vi "Microwave Amplifier Control Panel.vi"() -> ()   [LabVIEW 2009]
panel:
  in  "?":bool
  in  "?":bool
  out "Gain":dbl
  out "Forward Power":dbl
  out "Backwards Power":dbl
  in  "Set Gain":dbl
  in  "Operate":bool
  # "Microwave Amplifier"
  # "dBm"
  # "Watts"
  # "dBm"
  # "Watts"
  # "Standby"
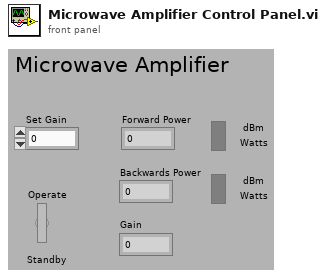
[diagram p1: front panel]
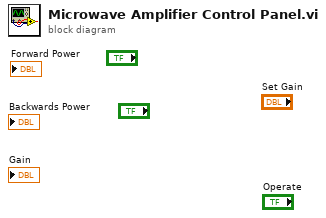
[diagram p0: block diagram]
diagram:
